vi "Update Calibration Example.vi"() -> ()   [LabVIEW 2020]
uses:
  <vilib>/Skyline/Configuration/Configuration HTTP_class/NI Skyline Configuration HTTP.lvclass/NI Skyline Configuration HTTP.ctl
  <vilib>/Skyline/Configuration/Configuration HTTP_class/Open Configuration HTTP.vi
  <vilib>/Skyline/Configuration/HTTP/Open Configuration (Desktop).vi
  <vilib>/Skyline/Configuration/Configuration HTTP_class/NI Skyline Configuration HTTP.lvclass
  <vilib>/Skyline/Configuration/Configuration_class/NI Skyline Configuration.lvclass
panel:
  in  "Temperature Sensors":cluster{"name":string, "reading":dbl}[](array[cluster]) {"reading" format="%#.2g"}
  in  "Calibration Date":timestamp format="%<%x>T"
  in  "Serial Number":string="012B6954"
  in  "Password":string="LabVIEW==="
  in  "Username":string="lvadmin"
  in  "Server":string="https://test.systemlink.io"
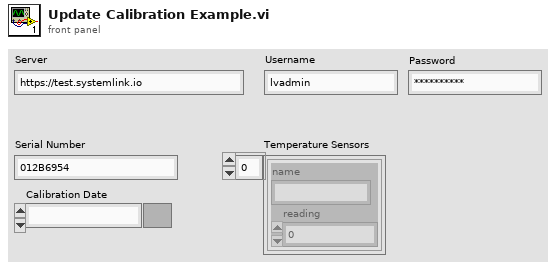
[diagram p1: front panel]
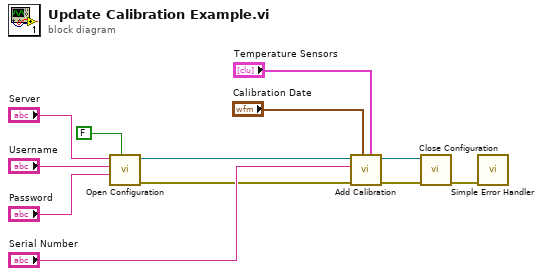
[diagram p0: block diagram]
diagram:
  n1 = call-poly <vilib>:"Open Configuration.vi"("verify server?"=FALSE, "password"="Password", "username"="Username", "server url"="Server") -> ("error out"=w6:errorcluster, "configuration"=w8:refnum<class "NI Skyline Configuration HTTP.lvclass">)  [unwired: 6 in]
  n2 = call "Add Calibration.vi"("Temperature Sensors"="Temperature Sensors", "Calibration Date"="Calibration Date", "error in"=w6, "Serial Number"="Serial Number", "NI Skyline Configuration HTTP in"=w8) -> ("error out"=w4:errorcluster, "NI Skyline Configuration HTTP out"=w5:refnum<class "NI Skyline Configuration HTTP.lvclass">)  [unwired: 5 in]
  n3 = call-dynamic "Close Configuration.vi"("error in (no error)"=w4, "configuration"=w5) -> ("error out"=w1:errorcluster)  [unwired: 9 in]
  n4 = call <vilib>:"Simple Error Handler.vi"("error in (no error)"=w1) -> ()  [unwired: 4 in, 5 out]
